vi "Get_Spect.vi"(8 "error in (no error)":errorcluster, 11 "Instruments in":refnum<class "Instruments.lvclass">) -> (0 "error out":errorcluster, 1 "Data":cluster{"Wavelength":dbl[], "EL Spectrum":dbl[]}, 2 "Graph":T1(array[cluster]), 3 "Instruments out":refnum<class "Instruments.lvclass">)   [LabVIEW 2012, in "Instruments.lvclass"]
uses:
  Instruments.lvclass
  Instruments.lvclass/Instruments.ctl
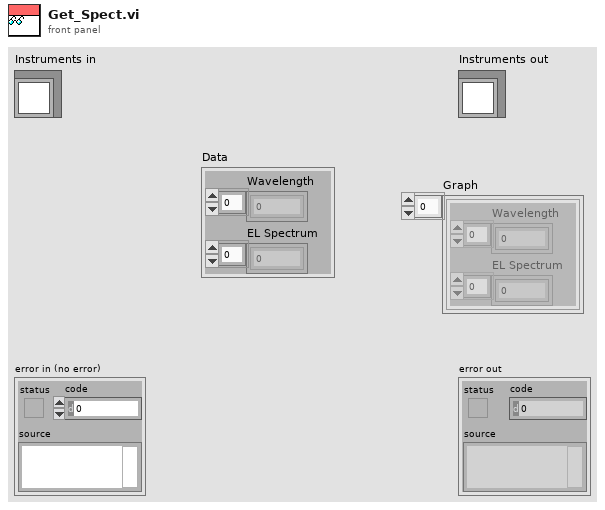
[diagram p1: front panel]
types:
  T1 = cluster{"Wavelength":dbl[], "EL Spectrum":dbl[]}[]
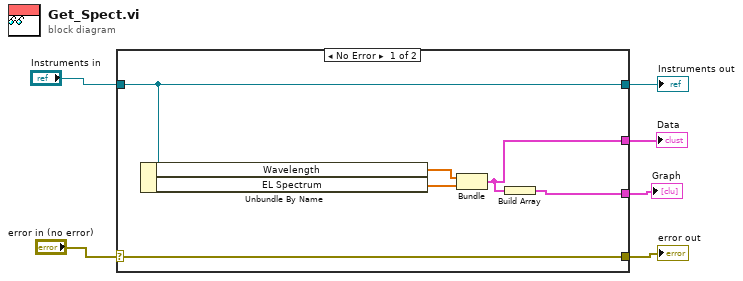
[diagram p0: block diagram]
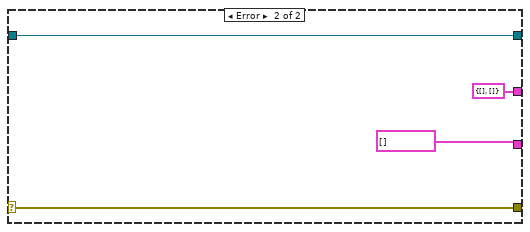
[diagram p2: hidden frame]
diagram:
  n1 = case shown="No Error" "error in (no error)" {
    selector: "error in (no error)" -> [w12 w15]
    tunnel: [w12 w15] -> w5
    tunnel: [w11 w16] -> w3
    tunnel: "Instruments in" -> [w11 w16]
    tunnel: [w8 T1 [] ("appended array")] -> w2
    tunnel: [w7 cluster{"Wavelength":dbl[], "EL Spectrum":dbl[]} {"Wavelength"=[], "EL Spectrum"=[]}] -> w1
    frame No Error {
      n2 = Unbundle By Name(w11) -> ("Wavelength"=w10:dbl[], "EL Spectrum"=w9:dbl[])
      n3 = Bundle("Wavelength"=w10, "EL Spectrum"=w9) -> (w7:cluster{"Wavelength":dbl[], "EL Spectrum":dbl[]})  [unwired: 1 in]
      n4 = Build Array(w7) -> (w8:T1)
    }
    frame Error {
    }
  }
  "error out" <- w5
  "Instruments out" <- w3
  "Graph" <- w2
  "Data" <- w1
